vi "Determine Clicked Array Element Index - Determine if Item Clicked.vi"(0 "Array Reference":refnum<vi>, 1 "Un-gapped left coordinates":i32[](array[numeric]), 2 "Minimal Array Properties.Bounds":T2, 3 "Minimal Array Properties.Position":T1, 4 "Coords of Click":T3, 5 "error in (no error)":errorcluster, 6 "Select Item":T4(ring)) -> (11 "Item Clicked?":bool, 13 "Item Visible?":bool, 14 "dup Array Reference":refnum<vi>, 15 "dup Un-gapped left coordinates":i32[](array[numeric]), 16 "dup Minimal Array Properties.Bounds":T2, 17 "dup Minimal Array Properties.Position":T1, 18 "dup Coords of Click":T3, 19 "error out":errorcluster)   [LabVIEW 2020]
doc: "Determine Clicked Array Element Index - Determine if Item Clicked.vi\n\nDescription:\nThis VI determines if the item specified by the Select Item input was clicked.\n\nInputs:\nArray Reference - Reference to the array to operate on.\n\nUn-gapped left coordinates - The left coordinates of each column with no element gap accounted for.\n\nMinimal Array Property.Bounds - Bounds property when the scrollbars, index display, label and caption are hidden.\n\nMinimal Array Property.Position - Position property when the scrollbars, index display, label and caption are hidden.\n\nCoords of Click - The screen coordinates of the click within the array. These values are used to determine if the click occurred on the selected item.\n\nSelect Item - Specifies the item to operate on.\n\nerror in - Standard error cluster.\n\nOutputs:\ndup Array Reference - Dup reference to the array to operate on.\n\ndup Un-gapped left coordinates - Dup left coordinates of each column with no element gap accounted for.\n\ndup Minimal Array Property.Bounds - Dup bounds property when the scrollbars, index display, label and caption are hidden.\n\ndup Minimal Array Property.Position - Dup position property when the scrollbars, index display, label and caption are hidden.\n\ndup Coords of Click - Dup screen coordinates of the click within the array. These values are used to determine if the click occurred on the selected item.\n\nerror out - standard error cluster.\n\nDeveloped By:\nMark.ridgley\nMark.Ridgley_LabVIEW.Developer@comcast.net"
uses:
  <vilib>/Utility/miscctls.llb/LVPoint32TypeDef.ctl
  <vilib>/Utility/miscctls.llb/LVBoundsTypeDef.ctl
  <vilib>/Utility/miscctls.llb/LVPositionTypeDef.ctl
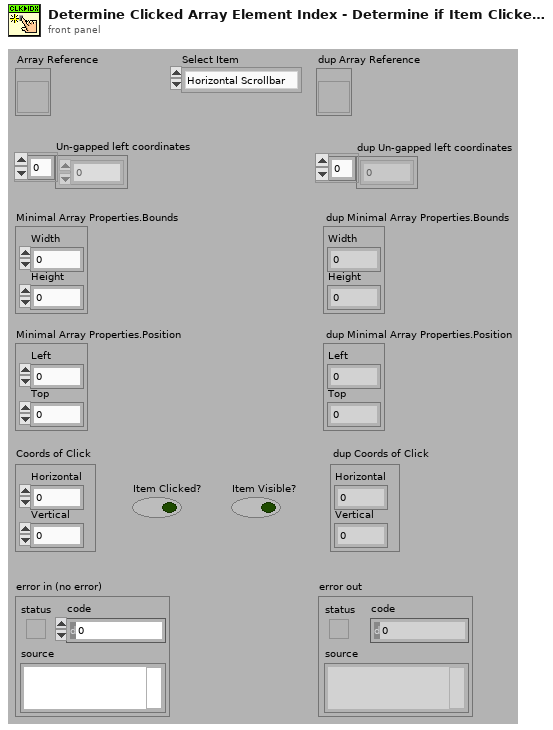
[diagram p1: front panel]
types:
  T1 = typedef "LVPositionTypeDef.ctl" = cluster{"Left":i32, "Top":i32}
  T2 = typedef "LVBoundsTypeDef.ctl" = cluster{"Width":u32, "Height":u32}
  T3 = typedef "LVPoint32TypeDef.ctl" = cluster{"Horizontal":i32, "Vertical":i32}
  T4 = enum16{"Horizontal Scrollbar", "Vertical Scrollbar", "Index Display"}
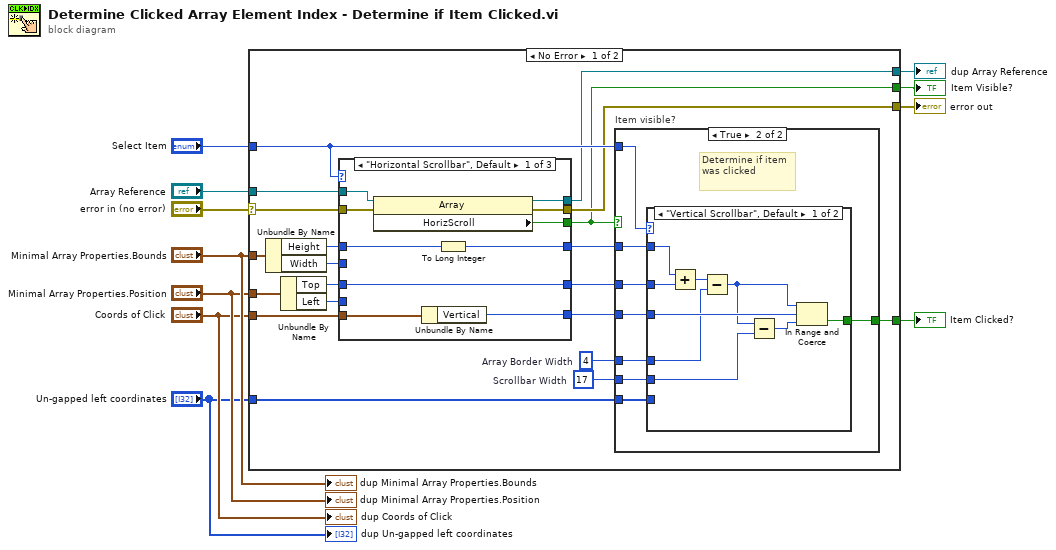
[diagram p0: block diagram]
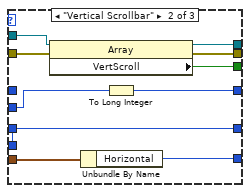
[diagram p2: hidden frame]
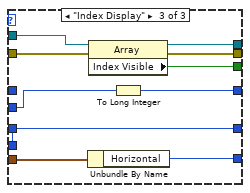
[diagram p3: hidden frame]
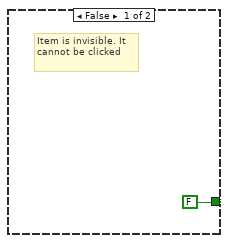
[diagram p4: hidden frame]
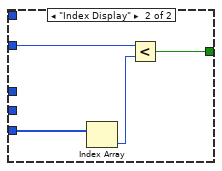
[diagram p5: hidden frame]
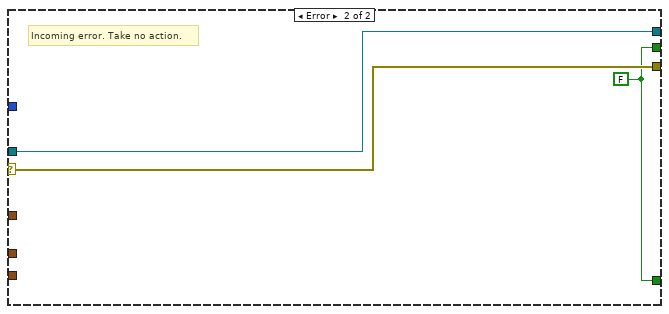
[diagram p6: hidden frame]
diagram:
  n1 = case shown="No Error" "error in (no error)" {
    selector: "error in (no error)" -> [w21 w86]
    tunnel: [w30 w84] -> w11
    tunnel: "Select Item" -> [w31 _]
    tunnel: "Coords of Click" -> [w27 _]
    tunnel: "Array Reference" -> [w26 w85]
    tunnel: [w25 w85] -> w8
    tunnel: [w24 w86] -> w7
    tunnel: [w22 w84] -> w6
    tunnel: "Un-gapped left coordinates" -> [w20 _]
    tunnel: "Minimal Array Properties.Bounds" -> [w16 _]
    tunnel: "Minimal Array Properties.Position" -> [w19 _]
    frame No Error {
      w29 = 4  # Array Border Width
      w28 = 17  # Scrollbar Width
      n2 = Unbundle By Name(w16) -> ("Height"=w15:u32, "Width"=w14:u32)
      n3 = Unbundle By Name(w19) -> ("Top"=w18:i32, "Left"=w17:i32)
      n4 = case shown="\"Horizontal Scrollbar\", Default" w31 {
        tunnel: w27 -> [w41 w51 w61]
        tunnel: [w40 w50 w60] -> w13
        tunnel: w26 -> [w39 w49 w59]
        tunnel: [w38 w48 w58] -> w25
        tunnel: [w37 w47 w57] -> w24
        tunnel: w21 -> [w36 w46 w56]
        tunnel: [w32 w42 w52] -> w23
        tunnel: [w34 w44 w53] -> w12
        tunnel: [w35 w45 w55] -> w22
        tunnel: w14 -> [_ w43 w54]
        tunnel: w17 -> [_ w44 w53]
        tunnel: w18 -> [w34 _ _]
        tunnel: w15 -> [w33 _ _]
        frame "Horizontal Scrollbar", Default {
          n5 = property class="Array"(reference=w39, error in=w36) -> (reference out=w38:refnum<vi>, error out=w37:errorcluster, "HorizScroll"=w35:bool)
          n6 = Unbundle By Name(w41) -> ("Vertical"=w40:i32)
          n7 = To Long Integer(number=w33) -> (32bit integer=w32:i32)
        }
        frame "Vertical Scrollbar" {
          n8 = property class="Array"(reference=w49, error in=w46) -> (reference out=w48:refnum<vi>, error out=w47:errorcluster, "VertScroll"=w45:bool)
          n9 = Unbundle By Name(w51) -> ("Horizontal"=w50:i32)
          n10 = To Long Integer(number=w43) -> (32bit integer=w42:i32)
        }
        frame "Index Display" {
          n11 = Unbundle By Name(w61) -> ("Horizontal"=w60:i32)
          n12 = property class="Array"(reference=w59, error in=w56) -> (reference out=w58:refnum<vi>, error out=w57:errorcluster, "Index Visible"=w55:bool)
          n13 = To Long Integer(number=w54) -> (32bit integer=w52:i32)
        }
      }
      n14 = case "Item visible?" shown="True" w22 {
        tunnel: [FALSE w66] -> w30
        tunnel: w23 -> [_ w70]
        tunnel: w13 -> [_ w69]
        tunnel: w29 -> [_ w68]
        tunnel: w28 -> [_ w67]
        tunnel: w12 -> [_ w65]
        tunnel: w31 -> [_ w64]
        tunnel: w20 -> [_ w63]
        frame False {
          # "Item is invisible. It cannot be clicked"
        }
        frame True {
          # "Determine if item\nwas clicked"
          n15 = case shown="\"Vertical Scrollbar\", Default" w64 {
            tunnel: w70 -> [w75 _]
            tunnel: w69 -> [w79 w80]
            tunnel: w68 -> [w74 _]
            tunnel: w67 -> [w73 _]
            tunnel: [w72 w82] -> w66
            tunnel: w65 -> [w71 _]
            tunnel: w63 -> [_ w81]
            frame "Vertical Scrollbar", Default {
              n16 = Add(x=w75, y=w71) -> (x+y=w76:i32)
              n17 = Subtract(x=w76, y=w74) -> (x-y=w77:i32)
              n18 = Subtract(x=w77, y=w73) -> (x-y=w78:i32)
              n19 = In Range and Coerce(upper limit=w77, x=w79, lower limit=w78) -> (In Range?=w72:bool)  [unwired: 1 out]
            }
            frame "Index Display" {
              n20 = Index Array(array=w81) -> (element=w83:i32)  [unwired: 1 in]
              n21 = Less?(x=w80, y=w83) -> (x < y?=w82:bool)
            }
          }
        }
      }
    }
    frame Error {
      w84 = FALSE ("VertScroll")
      # "Incoming error. Take no action."
    }
  }
  "Item Clicked?" <- w11
  "Item Visible?" <- w6
  "dup Array Reference" <- w8
  "error out" <- w7
  "dup Coords of Click" <- "Coords of Click"
  "dup Minimal Array Properties.Position" <- "Minimal Array Properties.Position"
  "dup Minimal Array Properties.Bounds" <- "Minimal Array Properties.Bounds"
  "dup Un-gapped left coordinates" <- "Un-gapped left coordinates"
